vi "Pulse DC Current.vi"(8 "error in (no error)":errorcluster, 10 "Params":variant, 11 "Source Measure Unit in":refnum<class "Source Measure Unit.lvclass">) -> (0 "error out":errorcluster, 3 "Source Measure Unit out":refnum<class "Source Measure Unit.lvclass">)   [LabVIEW 2020, in "Instrument.lvlib" / "Source Measure Unit.lvclass"]
uses:
  Source Measure Unit.lvclass
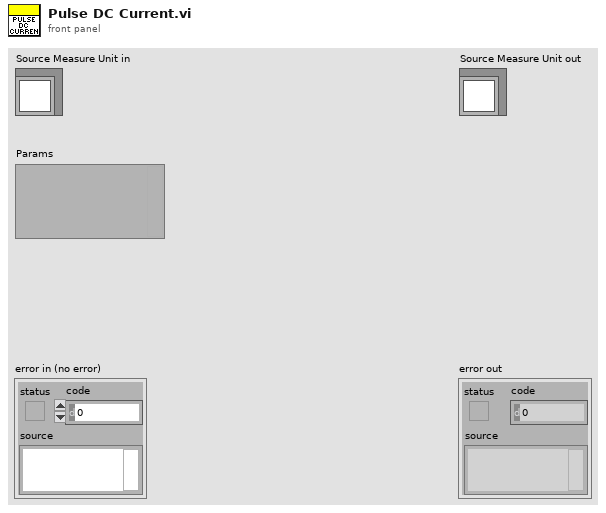
[diagram p1: front panel]
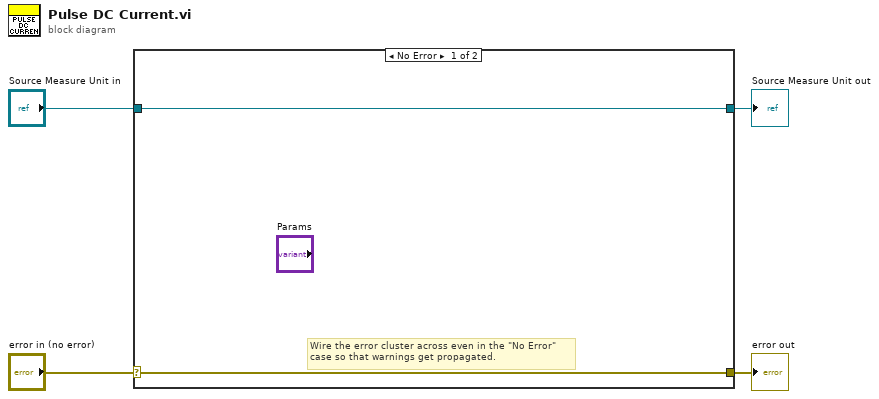
[diagram p0: block diagram]
diagram:
  n1 = case shown="No Error" "error in (no error)" {
    selector: "error in (no error)" -> [w5 w8]
    tunnel: [w5 w8] -> w3
    tunnel: [w6 w7] -> w1
    tunnel: "Source Measure Unit in" -> [w6 w7]
    frame No Error {
      # "Wire the error cluster across even in the \"No Error\"\ncase so that warnings get propagated."
    }
    frame Error {
    }
  }
  "error out" <- w3
  "Source Measure Unit out" <- w1
